vi "Diagnostic Sample.vi"(8 "error in (no error)":errorcluster, 10 "Acquisition Data":T1, 11 "MSX-E3711 in":refnum<class "MSX-E3711.lvclass">) -> (0 "error out":errorcluster, 2 "Acquisition Data Out":T1, 3 "MSX-E3711 out":refnum<class "MSX-E3711.lvclass">)   [LabVIEW 2014, in "MSX-E3711.lvlib" / "MSX-E3711.lvclass"]
uses:
  MSX-E3711.lvclass
  DriverMasterSync/build/DriverMasterSync.lvlibp/APIs/Data Queue/Acquisition Data Cluster.ctl
  DriverMasterSync/build/DriverMasterSync.lvlibp/APIs/Data Queue/Acquisition Data 1 Sample Cluster.ctl
  MSX-E3711.lvclass/MSX-E3711.ctl
  DriverMasterSync/build/DriverMasterSync.lvlibp/Modules/HAL/DriverMasterSync/DriverMasterSyncClass/DriverMasterSync.lvclass
  DriverMasterSync/build/DriverMasterSync.lvlibp/APIs/Data Queue/WINFAS 2 Data Queue.lvlib
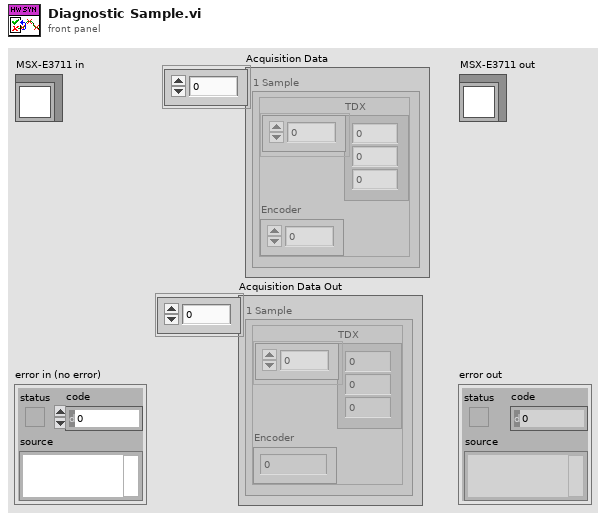
[diagram p1: front panel]
types:
  T1 = typedef "DriverMasterSync.lvlibp/WINFAS 2 Data Queue.lvlib/Acquisition Data Cluster.ctl" = T2[]
  T2 = typedef "DriverMasterSync.lvlibp/WINFAS 2 Data Queue.lvlib/Acquisition Data 1 Sample Cluster.ctl" = cluster{"TDX":sgl[], "Encoder":sgl}
  T3 = typedef "DriverMasterSync.lvlibp/HAL Config Data.ctl" = cluster{"HWSync Index":u32, "Driver Name":string, "Channel Mask":u64}
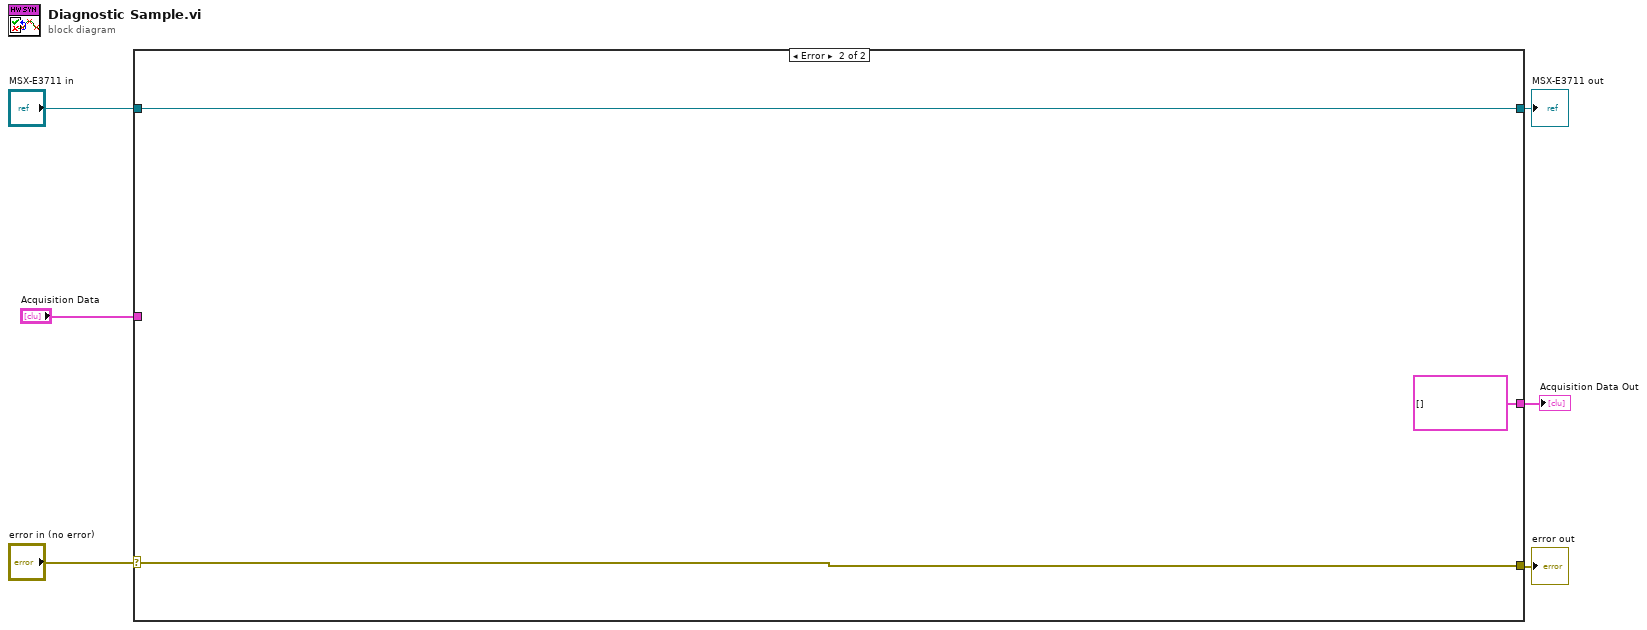
[diagram p0: block diagram]
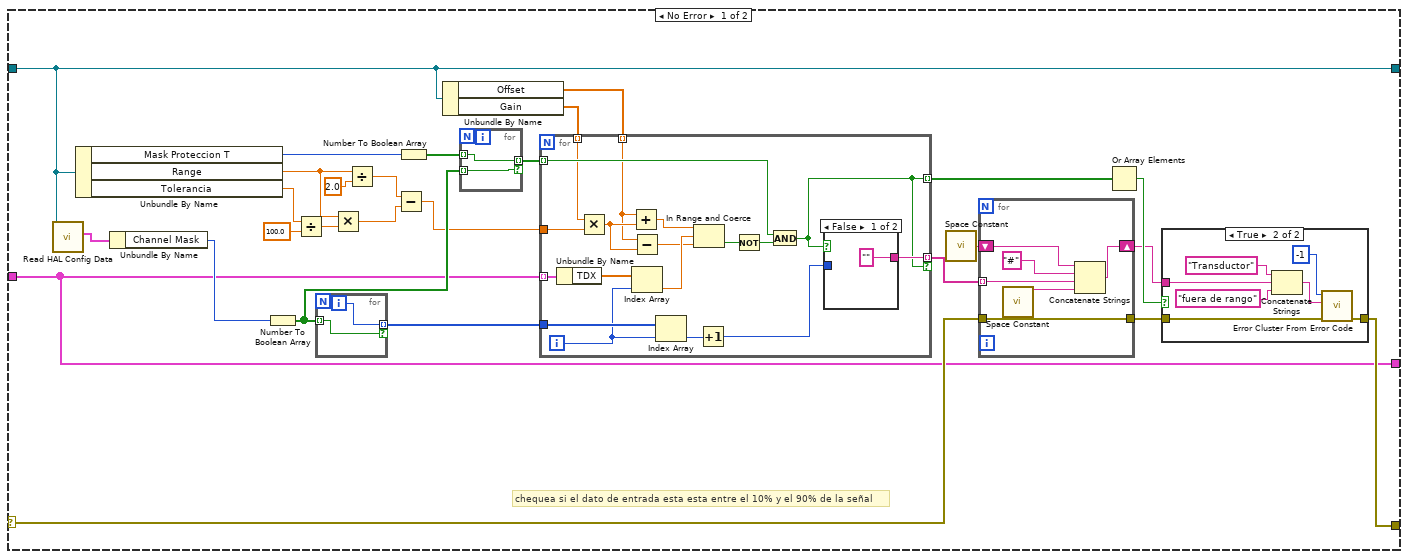
[diagram p2: hidden frame]
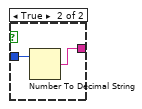
[diagram p4: hidden frame]
diagram:
  n1 = case shown="Error" "error in (no error)" {
    selector: "error in (no error)" -> [w9 w75]
    tunnel: [w8 w75] -> w5
    tunnel: [w10 w74] -> w3
    tunnel: "MSX-E3711 in" -> [w10 w74]
    tunnel: "Acquisition Data" -> [w7 _]
    tunnel: [w7 T1 [] ("Acquisition Data")] -> w1
    frame No Error {
      # "chequea si el dato de entrada esta esta entre el 10% y el 90% de la señal"
      n2 = call "Read HAL Config Data.vi"("DriverMasterSync in"=w10) -> ("HAL Config Data"=w11:T3)  [unwired: 8 in, 2 out]
      n3 = Unbundle By Name(w10) -> ("Mask Proteccion T"=w21:u64, "Range"=w15:sgl, "Tolerancia"=w19:sgl)
      n4 = Unbundle By Name(w11) -> ("Channel Mask"=w20:u64)
      n5 = Number To Boolean Array(number=w20) -> (Boolean array=w22:bool[])
      n6 = Divide(x=w19, y=sgl 100.0) -> (x/y=w32:sgl)
      n7 = for {
        tunnel: w22 -> [w50] mode=indexing
        tunnel: [w51] -> w31 mode=indexing if=w50
        i -> [w51]
      }
      n8 = Multiply(x=w15, y=w32) -> (x*y=w14:sgl)
      n9 = Divide(x=w15, y=sgl 2.0) -> (x/y=w13:sgl)
      n10 = Subtract(x=w13, y=w14) -> (x-y=w12:sgl)
      n11 = Number To Boolean Array(number=w21) -> (Boolean array=w24:bool[])
      n12 = Unbundle By Name(w10) -> ("Offset"=w17:sgl[], "Gain"=w16:sgl[])
      n13 = for {
        tunnel: w24 -> [w35] mode=indexing
        tunnel: [w35] -> w23 mode=indexing if=w34
        tunnel: w22 -> [w34] mode=indexing
      }
      n14 = for {
        tunnel: w7 -> [w69] mode=indexing
        tunnel: w31 -> [w65]
        tunnel: w23 -> [w66] mode=indexing
        tunnel: [w60] -> w30 mode=indexing
        tunnel: [w61] -> w26 mode=indexing if=w60
        tunnel: w17 -> [w53] mode=indexing
        tunnel: w16 -> [w56] mode=indexing
        tunnel: w12 -> [w57]
        i -> [w64]
        n15 = Unbundle By Name(w69) -> ("TDX"=w68:sgl[])
        n16 = Multiply(x=w56, y=w57) -> (x*y=w54:sgl)
        n17 = Add(x=w53, y=w54) -> (x+y=w55:sgl)
        n18 = Subtract(x=w53, y=w54) -> (x-y=w52:sgl)
        n19 = Index Array(array=w68, index=w64) -> (element=w67:sgl)
        n20 = Index Array(array=w65, index=w64) -> (element=w63:i32)
        n21 = In Range and Coerce(upper limit=w55, x=w67, lower limit=w52) -> (In Range?=w59:bool)  [unwired: 1 out]
        n22 = Increment(x=w63) -> (x+1=w62:i32)
        n23 = Not(x=w59) -> (.not. x?=w58:bool)
        n24 = And(x=w66, y=w58) -> (x .and. y?=w60:bool)
        n25 = case shown="False" w60 {
          tunnel: ["" w72] -> w61
          tunnel: w62 -> [_ w71]
          frame False {
          }
          frame True {
            n26 = Number To Decimal String(number=w71) -> (decimal integer string=w72:string)  [unwired: 1 in]
          }
        }
      }
      n27 = call <vilib>:"Space Constant.vi"() -> ("String"=w25:string)
      n28 = for {
        tunnel: [w41] -> w28
        tunnel: w9 -> [w41]
        shift-right: [w40] -> w27
        shift-left: w25 -> [w39]
        tunnel: w26 -> [w36] mode=indexing
        n29 = call <vilib>:"Space Constant.vi"() -> ("String"=w37:string)
        n30 = Concatenate Strings(w39, "#" ("string"), w36, w37) -> (w40:string)
      }
      n31 = Or Array Elements(Boolean array=w30) -> (logical OR=w29:bool)
      n32 = case shown="True" w29 {
        tunnel: [w42 w49] -> w8
        tunnel: w28 -> [w42 w44]
        tunnel: w27 -> [_ w43]
        frame False {
        }
        frame True {
          n33 = Concatenate Strings("Transductor", w43, "fuera de rango" ("string")) -> (w46:string)
          n34 = call <vilib>:"Error Cluster From Error Code.vi"("error in (no error)"=w44, "error message (\"\")"=w46, "error code (0)"=-1) -> ("error out"=w49:errorcluster)  [unwired: 6 in]
        }
      }
    }
    frame Error {
    }
  }
  "error out" <- w5
  "MSX-E3711 out" <- w3
  "Acquisition Data Out" <- w1
